vi "TimConstant.vi"() -> ()   [LabVIEW 2014]
uses:
  <userlib>/Nanonis Prog Interface V5/Nanonis Prog Interface.lvlib
panel:
  in  "stop":bool
  in  "Time constant":dbl format="%#_6p"
  in  "Low Pass":dbl
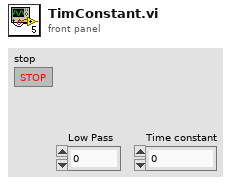
[diagram p1: front panel]
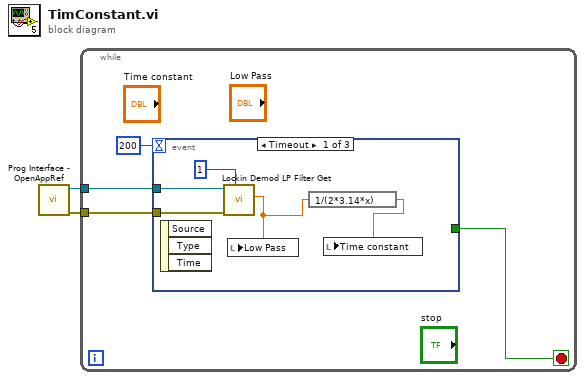
[diagram p0: block diagram]
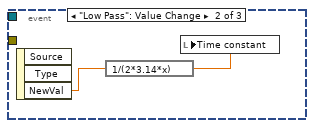
[diagram p2: hidden frame]
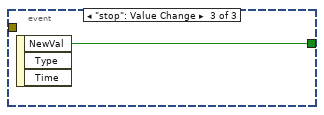
[diagram p3: hidden frame]
diagram:
  n1 = call <userlib>:"Prog Interface - OpenAppRef.vi"() -> ("Error out"=w1:errorcluster, "Application reference"=w2:refnum<vi>)  [unwired: 6 in]
  n2 = while {
    tunnel: w2 -> [w5]
    tunnel: w1 -> [w4]
    stop <- w3 stop-if-true
    n3 = event shown="[0] Timeout" {
      selector: _ -> [_ _ _]
      dyn-events: _ -> [_ _ _]
      timeout: 200 -> [_ _ _]
      tunnel: w5 -> [w11 _ _]
      tunnel: w4 -> [w10 _ _]
      tunnel: [_ _ w14] -> w3
      event Timeout {
        n4 = event-data() -> ()  [unwired: 1 in, 3 out]
        n5 = call <userlib>:"Lockin Demod LP Filter Get.vi"("Demodulator Index (1)"=1, "Error in (no error)"=w10, "Application ref in"=w11) -> ("LP Cutoff Frq (Hz)"=w8:sgl)  [unwired: 5 in, 3 out]
        n6 = local write "Low Pass"(w8) -> ()
        n7 = expression code="1/(2*3.14*x)"(w8) -> (w7:sgl)
        n8 = local write "Time constant"(w7) -> ()
      }
      event "Low Pass": Value Change {
        n9 = event-data() -> ("NewVal"=w13:dbl)  [unwired: 1 in, 2 out]
        n10 = expression code="1/(2*3.14*x)"(w13) -> (w12:dbl)
        n11 = local write "Time constant"(w12) -> ()
      }
      event "stop": Value Change {
        n12 = event-data() -> ("NewVal"=w14:bool)  [unwired: 1 in, 2 out]
      }
    }
  }
